vi "Home.vi"(8 "error in (no error)":errorcluster, 10 "Axes":T1={"X"=TRUE, "Y"=TRUE, "Z"=TRUE}, 11 "VISA resource name":refnum<visa-resource-name>) -> (0 "error out":errorcluster, 3 "VISA resource name out":refnum<visa-resource-name>)   [LabVIEW 2023, in "Marlin Instrument Driver.lvlib"]
doc: "Returns the current state of the configured X, Y, Z endstops. Takes into account any 'inverted endstop' settings, so one can confirm that the machine is interpreting the endstops correctly."
uses:
  Marlin Instrument Driver.lvlib
  controls/axes.ctl
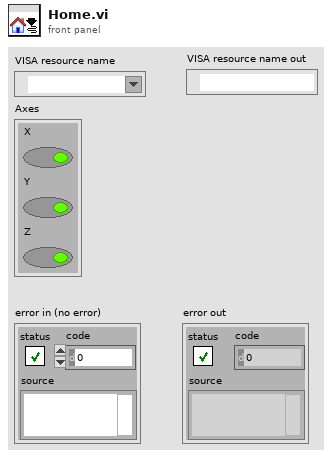
[diagram p1: front panel]
types:
  T1 = typedef "Marlin Instrument Driver.lvlib/axes.ctl" = cluster{"X":bool, "Y":bool, "Z":bool}
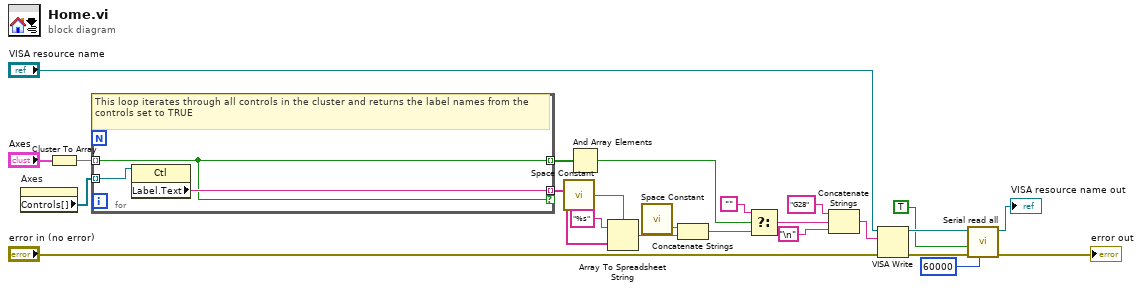
[diagram p0: block diagram]
diagram:
  n1 = property on="Axes" class="Clust (strict)"() -> ("Controls[]"=w14:refnum<vi>[])  [unwired: 2 in, 2 out]
  n2 = Cluster To Array(cluster="Axes") -> (array=w12:bool[])
  n3 = for {
    tunnel: w14 -> [w27] mode=indexing
    tunnel: w12 -> [w25] mode=indexing
    tunnel: [w26] -> w10 mode=indexing if=w25
    tunnel: [w25] -> w11 mode=indexing
    # "This loop iterates through all controls in the cluster and returns the label names from the controls set to TRUE"
    n4 = property class="Ctl"(reference=w27) -> ("Label.Text"=w26:string)  [unwired: 1 in, 2 out]
  }
  n5 = call <vilib>:"Space Constant.vi"() -> ("String"=w8:string)
  n6 = And Array Elements(Boolean array=w11) -> (logical AND=w7:bool)
  n7 = Array To Spreadsheet String(delimiter (Tab)=w8, array=w10, 3:"%s" ("format string")) -> (spreadsheet string=w4:string)
  n8 = call <vilib>:"Space Constant.vi"() -> ("String"=w2:string)
  n9 = Concatenate Strings(w2, w4) -> (w3:string)
  n10 = Select(t="", s=w7, f=w3) -> (s? t:f=w6:string)
  n11 = Concatenate Strings("G28" ("command"), w6, "\n") -> (w21:string)
  n12 = VISA Write(VISA resource name="VISA resource name", write buffer=w21, error in (no error)="error in (no error)") -> (VISA resource name out=w19:refnum<visa-resource-name>, error out=w20:errorcluster)  [unwired: 1 out]
  n13 = call "Serial read all.vi"("timeout (10000ms)"=u32 60000, "error in (no error)"=w20, "Wait for OK"=TRUE, "VISA Refnum in"=w19) -> ("error out"=→"error out":errorcluster, "VISA Refnum out"=→"VISA resource name out":refnum<visa-resource-name>)  [unwired: 4 in, 2 out]
